vi "Meas Proc QWTB Load Result Spectra.vi"(7 "phase ref":refnum<vi>, 8 "error in":errorcluster, 11 "meas root":path) -> (0 "error out":errorcluster, 3 "graphs":T1[](array[typedef]))   [LabVIEW 2018]
uses:
  Meas Proc QWTB Spectrum Data.ctl
  octave/infolib.lvlibp/Private/Get key polymorph parts/GetString.vi
  octave/infolib.lvlibp/Private/Get matrix polymorph parts/Get 1D String.vi
  octave/infolib.lvlibp/Private/Get key polymorph parts/GetI64.vi
  octave/infolib.lvlibp/Private/Get matrix polymorph parts/Get 2D String.vi
  octave/infolib.lvlibp
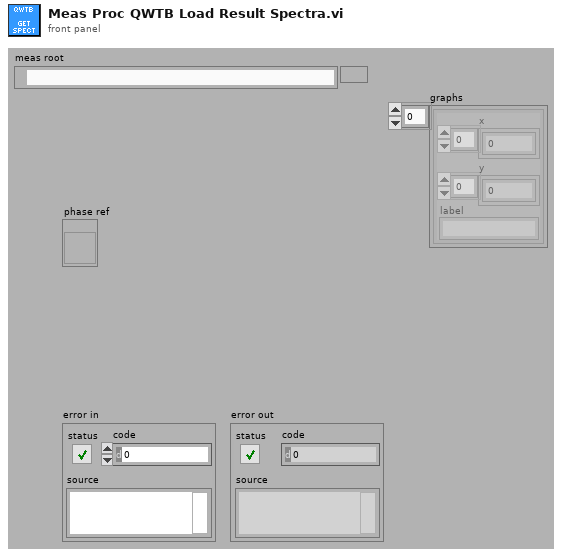
[diagram p1: front panel]
types:
  T1 = typedef "Meas Proc QWTB Spectrum Data.ctl" = cluster{"x":sgl[], "y":sgl[], "label":string}
  T2 = typedef "MAT Type Representation.ctl" = enum16{"DBL", "SGL", "I32", "I16", "U16", "U8", "CDB", "CSG", "STR"}
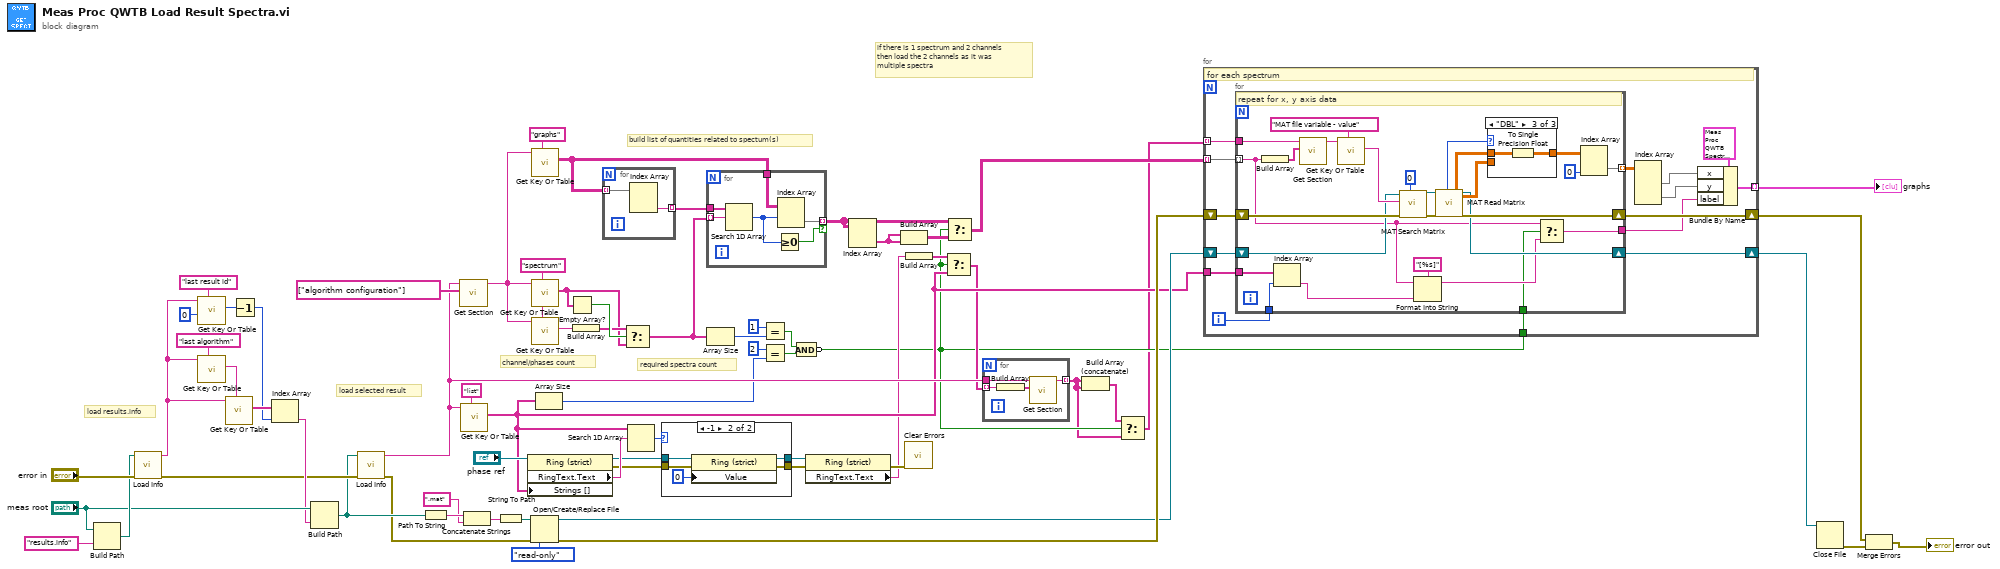
[diagram p0: block diagram]
diagram:
  w25 = "spectrum" ("key description")
  # "if there is 1 spectrum and 2 channels\nthen load the 2 channels as it was\nmultiple spectra"
  # "channel/phases count"
  # "required spectra count"
  # "load selected result"
  # "load results.info"
  # "build list of quantities related to spectum(s)"
  n1 = Build Path(base path="meas root", name or relative path="results.info") -> (appended path=w57:path)
  n2 = call "Load Info.vi"("error in"="error in", "filename"=w57) -> ("error out"=w54:errorcluster, "info data"=w62:string)  [unwired: 8 in]
  n3 = call-poly "Get Key Or Table.vi"("key description"="last result id", "numeric"=i64 0, "info data"=w62) -> ("value"=w60:i64)  [unwired: 5 in, 3 out]
  n4 = call-poly "Get Key Or Table.vi"("key description"="last algorithm", "info data"=w62) -> ("value"=w63:string)  [unwired: 6 in, 3 out]
  n5 = call-poly "Get Key Or Table.vi"("key description"=w63, "info data"=w62) -> ("value"=w61:string[])  [unwired: 6 in, 3 out]
  n6 = Decrement(x=w60) -> (x-1=w59:i64)
  n7 = Index Array(array=w61, index=w59) -> (element=w55:string)
  n8 = Build Path(base path="meas root", name or relative path=w55) -> (appended path=w39:path)
  n9 = call "Load Info.vi"("error in"=w54, "filename"=w39) -> ("error out"=w34:errorcluster, "info data"=w42:string)  [unwired: 8 in]
  n10 = Path To String(path=w39) -> (string=w38:string)
  n11 = call "Get Section.vi"("sections"=string[] ["algorithm configuration"], "info data"=w42) -> ("section part"=w24:string)  [unwired: 8 in, 1 out]
  n12 = call-poly "Get Key Or Table.vi"("key description"="list", "info data"=w42) -> ("value"=w8:string[])  [unwired: 6 in, 3 out]
  n13 = Concatenate Strings(w38, ".mat" ("name or relative path")) -> (w36:string)
  n14 = String To Path(string=w36) -> (path=w35:path)
  n15 = property class="Ring (strict)"(reference="phase ref", "Strings []"=w8) -> (reference out=w47:refnum<vi>, error out=w46:errorcluster, "RingText.Text"=w49:string)  [unwired: 1 in]
  n16 = Open/Create/Replace File(file path (use dialog)=w35, error in=w34, access (0:read/write)=enum16{"read/write", "read-only", "write-only"}."read-only") -> (refnum out=w30:refnum<file>, error out=w32:errorcluster)  [unwired: 3 in, 1 out]
  n17 = call-poly "Get Key Or Table.vi"("key description"="graphs", "info data"=w24) -> ("value"=w40:string[][])  [unwired: 6 in, 3 out]
  n18 = call-poly "Get Key Or Table.vi"("key description"=w25, "info data"=w24) -> ("value"=w20:string[])  [unwired: 6 in, 3 out]
  n19 = call-poly "Get Key Or Table.vi"("key description"=w25, "info data"=w24) -> ("value"=w22:string)  [unwired: 6 in, 3 out]
  n20 = Array Size(array=w8) -> (size(s)=w18:i32)
  n21 = Empty Array?(array=w20) -> (empty?=w23:bool)
  n22 = Build Array(w22) -> (w21:string[])
  n23 = for {
    tunnel: w40 -> [w69] mode=indexing
    tunnel: [w68] -> w41 mode=indexing
    n24 = Index Array(array=w69) -> (element #2=w68:string)  [unwired: 2 in, 1 out]
  }
  n25 = Select(t=w21, s=w23, f=w20) -> (s? t:f=w19:string[])
  n26 = Search 1D Array(1D array=w8, element=w49) -> (index of element=w48:i32)  [unwired: 1 in]
  n27 = case shown="-1" w48 {
    tunnel: w47 -> [w71 w76]
    tunnel: w46 -> [w70 w74]
    tunnel: [w70 w73] -> w45
    tunnel: [w71 w72] -> w44
    frame Default {
    }
    frame -1 {
      n28 = property class="Ring (strict)"(reference=w76, error in=w74, "Value"=u16 0) -> (reference out=w72:refnum<vi>, error out=w73:errorcluster)
    }
  }
  n29 = for {
    tunnel: w19 -> [w81] mode=indexing
    tunnel: w41 -> [w82]
    tunnel: w40 -> [w80]
    tunnel: [w79] -> w9 mode=indexing if=w78
    n30 = Search 1D Array(1D array=w82, element=w81) -> (index of element=w77:i32)  [unwired: 1 in]
    n31 = Greater Or Equal To 0?(x=w77) -> (x >= 0?=w78:bool)
    n32 = Index Array(array=w80, index (row)=w77) -> (element=w79:string[])  [unwired: 1 in]
  }
  n33 = Array Size(array=w19) -> (size(s)=w16:i32)
  n34 = Equal?(x=1, y=w16) -> (x = y?=w13:bool)
  n35 = Equal?(x=2, y=w18) -> (x = y?=w14:bool)
  n36 = Compound Arithmetic op=AND(w13, w14) -> (invert w4:bool)
  n37 = property class="Ring (strict)"(reference=w44, error in=w45) -> (error out=w43:errorcluster, "RingText.Text"=w7:string)  [unwired: 1 out]
  n38 = Index Array(array=w9) -> (element=w10:string[])  [unwired: 2 in]
  n39 = Build Array(w10, w10) -> (w12:string[][])
  n40 = call <vilib>:"Clear Errors.vi"("error in (no error)"=w43) -> ()  [unwired: 5 in, 2 out]
  n41 = Build Array(w7) -> (w6:string[])
  n42 = Select(t=w6, s=w4, f=w8) -> (s? t:f=w5:string[])
  n43 = Select(t=w9, s=w4, f=w12) -> (s? t:f=w11:string[][])
  n44 = for {
    tunnel: w5 -> [w86] mode=indexing
    tunnel: w42 -> [w84]
    tunnel: [w83] -> w2 mode=indexing
    n45 = Build Array(w86) -> (w85:string[])
    n46 = call "Get Section.vi"("sections"=w85, "info data"=w84) -> ("section part"=w83:string)  [unwired: 8 in, 1 out]
  }
  n47 = Build Array (concatenate)(w2, w2) -> (w3:string[])
  n48 = Select(t=w3, s=w4, f=w2) -> (s? t:f=w1:string[])
  n49 = for {
    tunnel: w11 -> [w101] mode=indexing
    tunnel: w1 -> [w100] mode=indexing
    shift-right: [w99] -> w26
    shift-left: w32 -> [w98]
    tunnel: [w94] -> w31 mode=indexing
    shift-right: [w90] -> w29
    shift-left: w30 -> [w91]
    tunnel: w8 -> [w88]
    tunnel: w4 -> [w87]
    i -> [w89]
    # "for each spectrum"
    n50 = for {
      tunnel: w101 -> [w103] mode=indexing
      tunnel: w100 -> [w127]
      shift-right: [w119] -> w99
      shift-left: w98 -> [w118]
      tunnel: [w112] -> w97 mode=indexing
      tunnel: [w109] -> w92
      shift-right: [w110] -> w90
      shift-left: w91 -> [w111]
      tunnel: w89 -> [w106]
      tunnel: w88 -> [w105]
      tunnel: w87 -> [w102]
      # "repeat for x, y axis data"
      n51 = Build Array(w103) -> (w126:string[])
      n52 = Index Array(array=w105, index=w106) -> (element=w104:string)
      n53 = call "Get Section.vi"("sections"=w126, "info data"=w127) -> ("section part"=w125:string)  [unwired: 8 in, 1 out]
      n54 = call-poly "Get Key Or Table.vi"("key description"="MAT file variable - value", "info data"=w125) -> ("value"=w123:string)  [unwired: 6 in, 3 out]
      n55 = call "MAT Search Matrix.vi"("offset in (-1: current position)"=i64 0, "Error In"=w118, "matrix name"=w123, "Ref Num"=w111) -> ("error out"=w121:errorcluster, "Dup Ref Num"=w120:refnum<file>)  [unwired: 6 in]
      n56 = Format Into String(format string="[%s]", initial string=w103, w104) -> (resulting string=w107:string)  [unwired: 1 in, 1 out]
      n57 = call "MAT Read Matrix.vi"("Ref Num"=w120, "Error In"=w121) -> ("Representation"=w117:T2, "DBL"=w115:dbl[][], "Dup Ref Num"=w110:refnum<file>, "SGL"=w116:sgl[][], "error out"=w119:errorcluster)  [unwired: 5 in, 8 out]
      n58 = case shown="\"DBL\"" w117 {
        tunnel: w116 -> [w128 _ _]
        tunnel: w115 -> [_ _ w130]
        tunnel: [w128 _ w129] -> w114
        frame "SGL" {
        }
        frame Default {
        }
        frame "DBL" {
          n59 = To Single Precision Float(number=w130) -> (single precision float=w129:sgl[][])
        }
      }
      n60 = Select(t=w103, s=w102, f=w107) -> (s? t:f=w109:string)
      n61 = Index Array(array=w114, index (col)=0 ("disabled index (col)")) -> (element=w112:sgl[])  [unwired: 1 in]
    }
    n62 = Index Array(array=w97) -> (element #1=w96:sgl[], element #2=w95:sgl[])  [unwired: 4 in]
    n63 = Bundle By Name(cluster=T1 {"x"=array[24001 elements], "y"=array[24001 elements], "label"=""} ("Meas Proc QWTB Spectrum Data"), "x"=w96, "y"=w95, "label"=w92) -> (w94:T1)
  }
  "graphs" <- w31
  n64 = Close File(refnum=w29) -> (error out=w28:errorcluster)  [unwired: 1 in, 1 out]
  n65 = Merge Errors(w26, w28) -> (→"error out":errorcluster)
